vi "LEBITplc.GetLastLoadedFiles.vi"(1 "GUINames":string[](array[string]), 4 "LLFLocation":string) -> (15 "GUINames":string[](array[string]), 16 "Last Loaded File Array":string[](array[string]), 18 "LLFLocation":string)   [LabVIEW 2014, in "LEBITplc.lvlib"]
uses:
  LEBITplc.lvlib
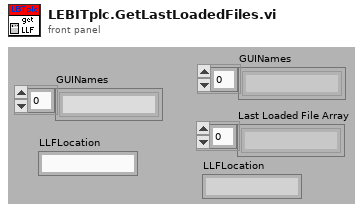
[diagram p1: front panel]
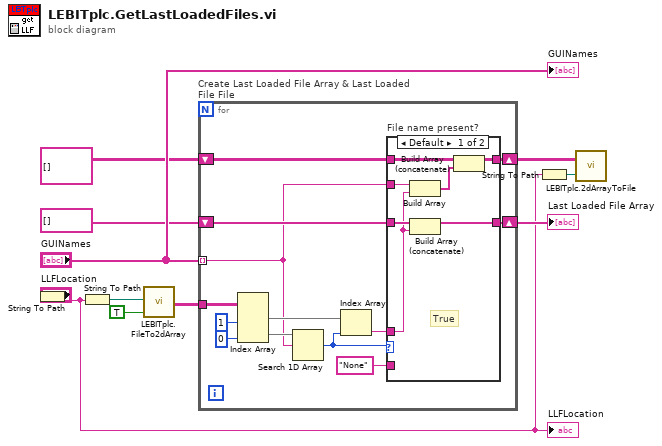
[diagram p0: block diagram]
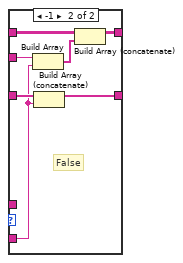
[diagram p2: hidden frame]
diagram:
  n1 = String To Path(string="LLFLocation") -> ()  [unwired: 1 out]
  n2 = String To Path(string="LLFLocation") -> (path=w7:path)
  n3 = call "LEBITplc.FileTo2dArray.vi"("file path (dialog if empty)"=w7, "Create if ness."=TRUE) -> ("Array"=w9:string[][])  [unwired: 16 in, 1 out]
  n4 = for "Create Last Loaded File Array & Last Loaded File File" {
    tunnel: "GUINames" -> [w14] mode=indexing
    tunnel: w9 -> [w23]
    shift-right: [w22] -> w8
    shift-left: string[] [] -> [w21]
    shift-right: [w15] -> w3
    shift-left: string[][] [] -> [w16]
    n5 = Index Array(array=w23, index (col) #1=1 ("disabled index (col)"), index (col) #2=0 ("index (col)")) -> (element #1=w18:string[], element #2=w17:string[])  [unwired: 2 in]
    n6 = Search 1D Array(1D array=w17, element=w14) -> (index of element=w12:i32)  [unwired: 1 in]
    n7 = Index Array(array=w18, index=w12) -> (element=w13:string)
    n8 = case "File name present?" shown="Default" w12 {
      tunnel: [w30 w37] -> w22
      tunnel: w21 -> [w29 w36]
      tunnel: w16 -> [w28 w35]
      tunnel: [w27 w34] -> w15
      tunnel: w14 -> [w25 w32]
      tunnel: w13 -> [w24 _]
      tunnel: "None" ("element") -> [_ w31]
      frame Default {
        # "True"
        n9 = Build Array(w25, w24) -> (w26:string[])
        n10 = Build Array (concatenate)(w29, w24) -> (w30:string[])
        n11 = Build Array (concatenate)(w28, w26) -> (w27:string[][])
      }
      frame -1 {
        # "False"
        n12 = Build Array(w32, w31) -> (w33:string[])
        n13 = Build Array (concatenate)(w36, w31) -> (w37:string[])
        n14 = Build Array (concatenate)(w35, w33) -> (w34:string[][])
      }
    }
  }
  "Last Loaded File Array" <- w8
  n15 = String To Path(string="LLFLocation") -> (path=w2:path)
  n16 = call "LEBITplc.2dArrayToFile.vi"("file path (dialog if empty)"=w2, "Array"=w3) -> ()  [unwired: 2 in]
  "GUINames" <- "GUINames"
  "LLFLocation" <- "LLFLocation"
